vi "ArduinoClose.vi"(8 "error in (no error)":errorcluster, 11 "ArduinoControl in":refnum<class "ArduinoControl.lvclass">) -> (0 "error out":errorcluster, 3 "ArduinoControl out":refnum<class "ArduinoControl.lvclass">)   [LabVIEW 2013, in "ArduinoControl.lvclass"]
uses:
  ArduinoControl.lvclass
  ArduinoControl.lvclass/ArduinoControl.ctl
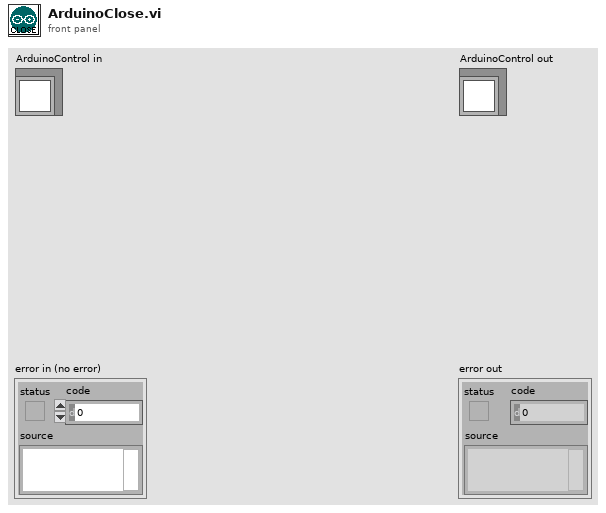
[diagram p1: front panel]
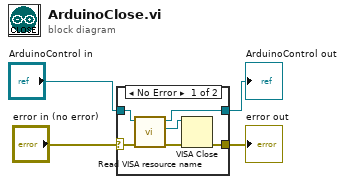
[diagram p0: block diagram]
diagram:
  n1 = case shown="No Error" "error in (no error)" {
    selector: "error in (no error)" -> [w8 w12]
    tunnel: [w5 w12] -> w3
    tunnel: [w9 w11] -> w1
    tunnel: "ArduinoControl in" -> [w10 w11]
    frame No Error {
      n2 = call "Read VISA resource name.vi"("error in (no error)"=w8, "ArduinoControl in"=w10) -> ("error out"=w6:errorcluster, "VISA resource name"=w7:refnum<visa-resource-name>, "ArduinoControl out"=w9:refnum<class "ArduinoControl.lvclass">)  [unwired: 7 in]
      n3 = VISA Close(VISA resource name=w7, error in (no error)=w6) -> (error out=w5:errorcluster)
    }
    frame Error {
    }
  }
  "error out" <- w3
  "ArduinoControl out" <- w1
